vi "BuildGrid.vi"(6 "Ygoal":dbl format="%#_13g", 7 "GridParameter":dbl, 8 "Ystart":dbl format="%#_13g", 9 "Xgoal":dbl format="%#_13g", 10 "Xstart":dbl format="%#_13g") -> (0 "Nó goal":dbl[](array[numeric]), 1 "ClosedSet out":dbl[][](array[numeric]), 2 "grid out":T1, 3 "Nó start":dbl[](array[numeric]))   [LabVIEW 2016]
uses:
  Core/AI Input.ctl
  Core/AI Robot.ctl
  Intel/Functions Enum.ctl
  Intel/AttackerStates.ctl
  Core/AI Ball.ctl
  Core/Field Size.ctl
  Core/AI Judge.ctl
  Intel/Command Enum.ctl
  Util/Events/Events.ctl
  grid.ctl
  elementGrid.ctl
panel:
  in  "y pai":dbl
  in  "x pai":dbl
  in  "id":dbl
  in  "G":dbl
  in  "H":dbl
  in  "F":dbl
  in  "dy 2":dbl[](array[numeric])=[1.0, -1.0, 0.0, 0.0, 1.0, -1.0, 1.0, -1.0]
  in  "dx 2":dbl[](array[numeric])=[0.0, 0.0, 1.0, -1.0, 1.0, 1.0, -1.0, -1.0]
  in  "dy":dbl[](array[numeric])=[1.0, -1.0, 0.0, 0.0, 1.0, -1.0, 1.0, -1.0]
  in  "dx":dbl[](array[numeric])=[0.0, 0.0, 1.0, -1.0, 1.0, 1.0, -1.0, -1.0]
  in  "IA State Input":T3={"our_robots"=[], "enemy_robots"=[], "balls"=[], "geometry"={"line_width"=0, "field_length"=0, "field_width"=0, "boundary_width"=0, "referee_width"=0, "goal_width"=0, "goal_depth"=0, "goal_wall_width"=0, "center_circle_radius"=0, "defense_radius"=0, "defense_stretch"=0, "free_kick_from_defense_dist"=0, "penalty_spot_from_field_line_dist"=0, "penalty_line_from_spot_dist"=0}, "IA Judge"={"stage"="", "command"="", "our_goalie_id"=0.0, "enemy_goalie_id"=0.0, "command enum"=enum."Halt", "Time"=enum."Azul"}, "Received Timestamp"=timestamp(0 s since 1904-01-01), "Events"={"Touch"=FALSE, "Ball out"=FALSE, "id touch"=0.0, "Ball out of \nVision"=FALSE, "Ball inside \nGoalie area"=FALSE, "Robot not responding"=FALSE, "Robots responding status"=[1.0, 1.0, 1.0, 1.0, 1.0, 1.0], "Enemy Ball \nPossession"=FALSE, "Pass State"=FALSE, "id end of pass"=0.0, "Kick"=FALSE, "Id ini Possession"=0.0, "Ball Possesion"=FALSE, "Id Possesion"=0.0}}
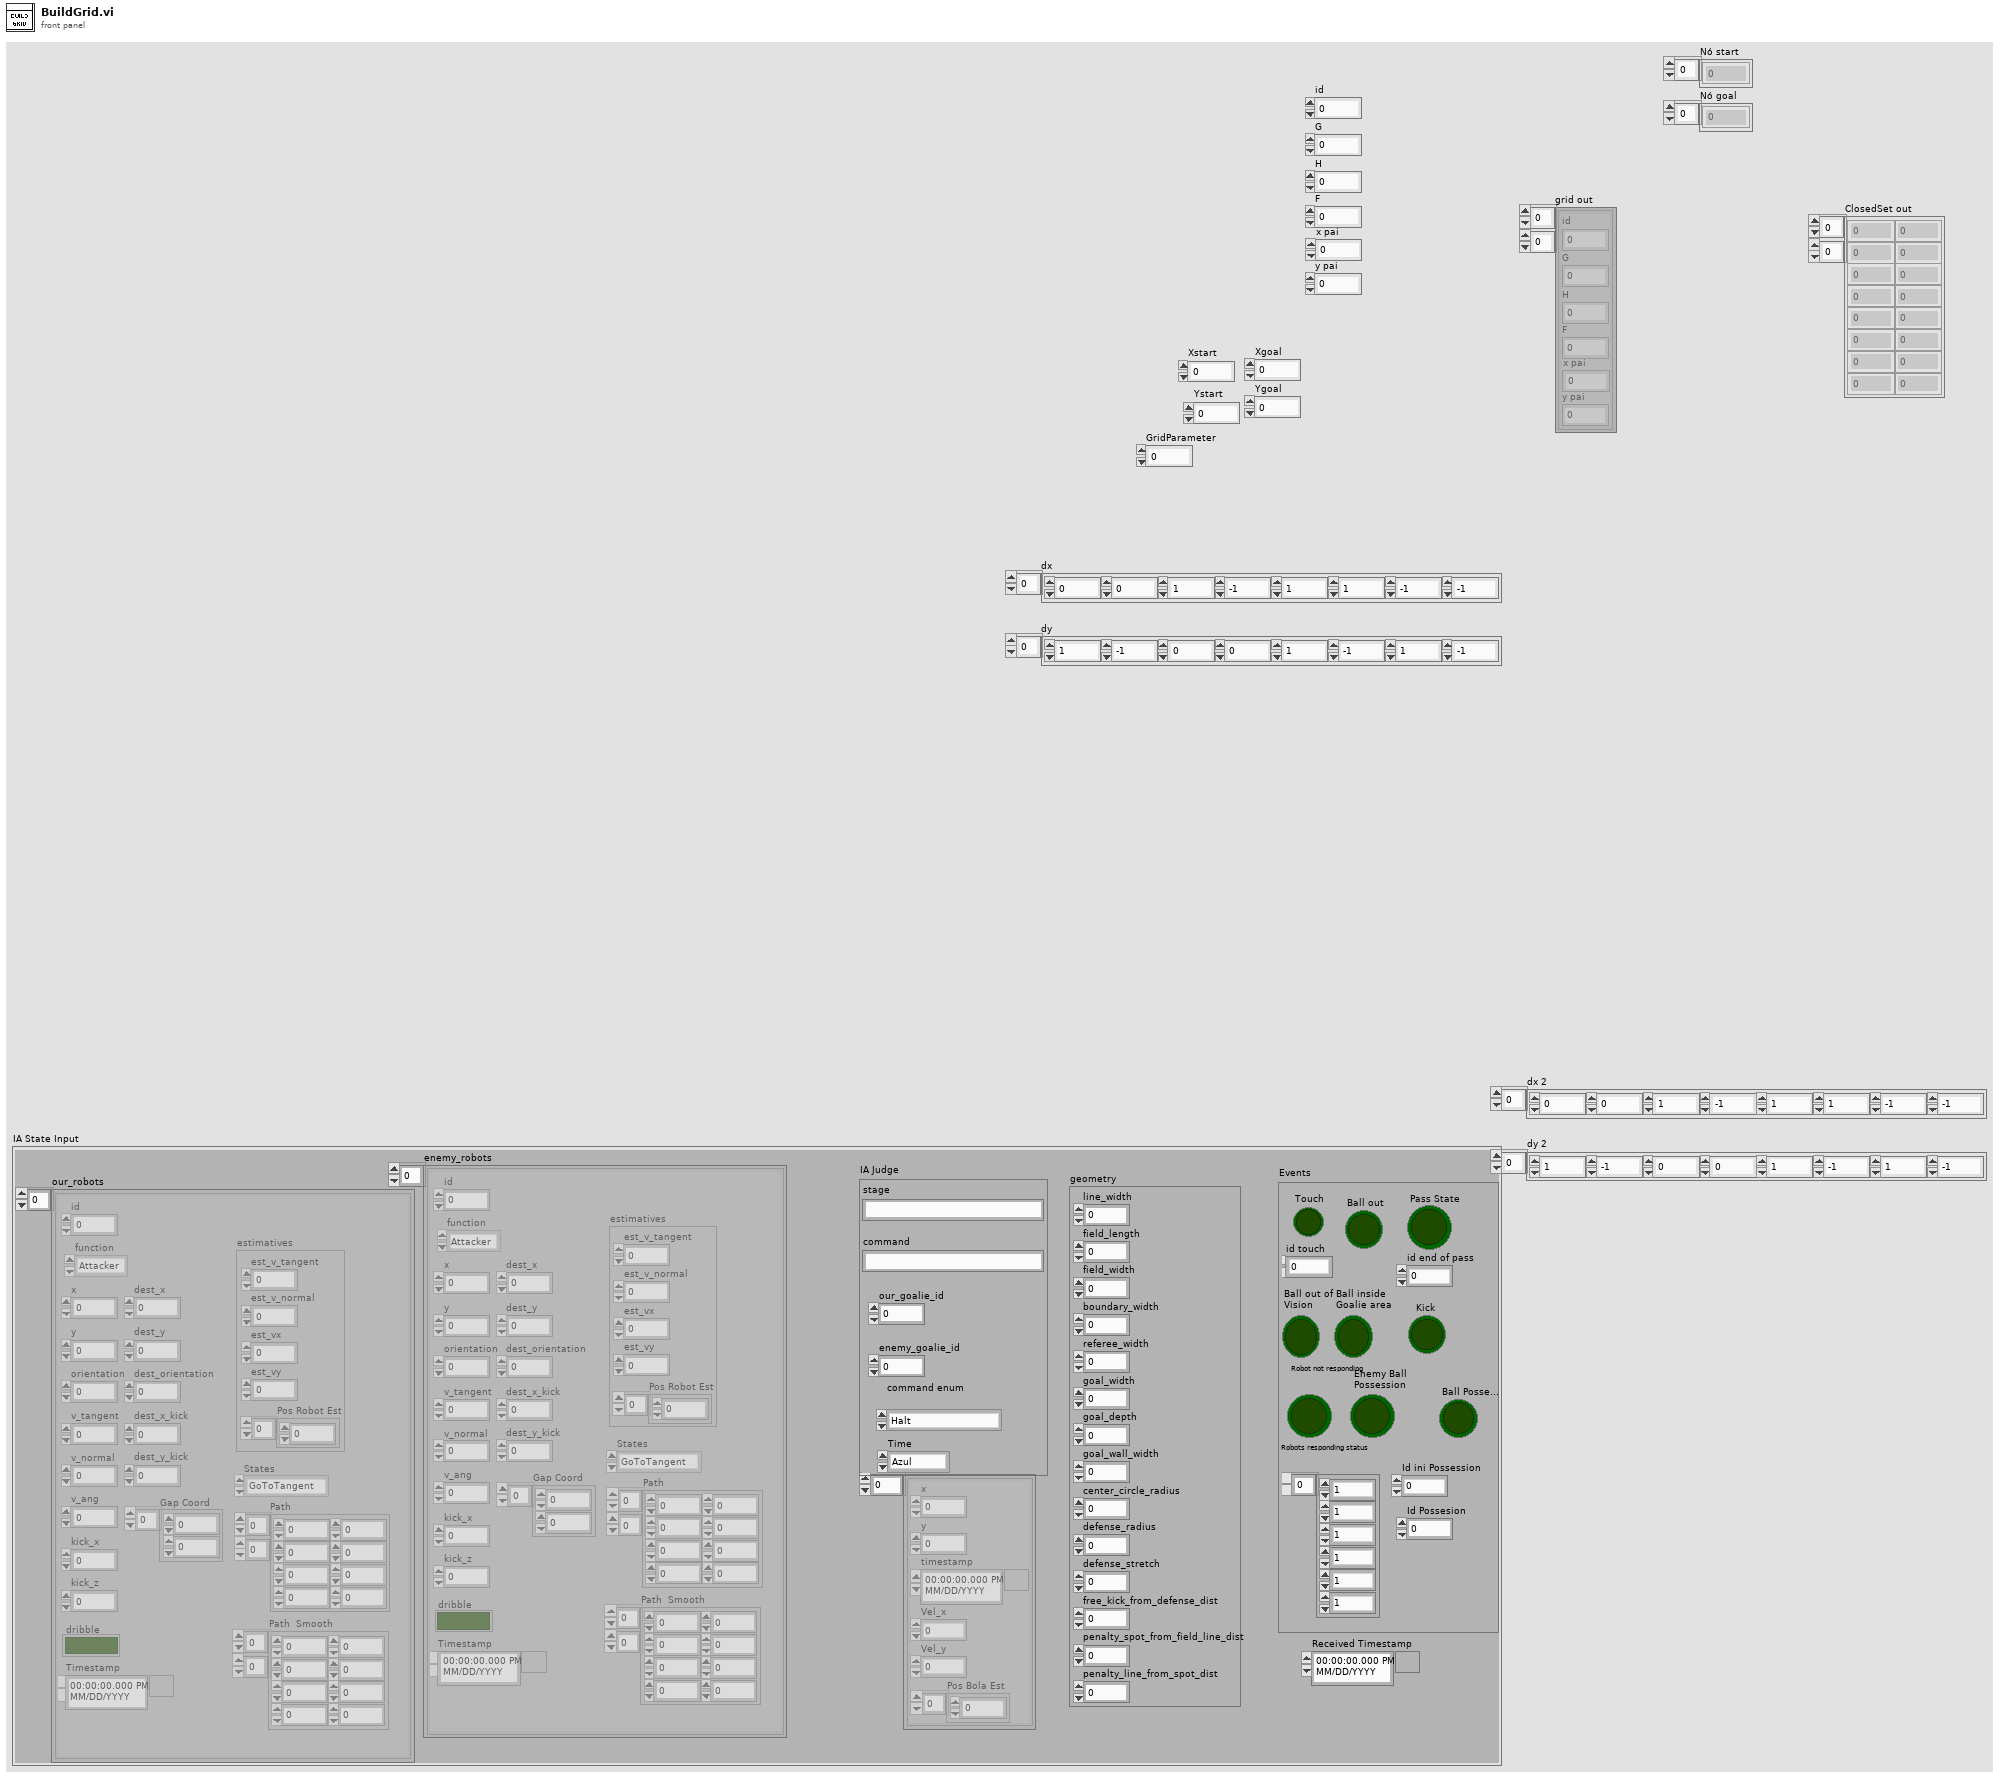
[diagram p1: front panel]
types:
  T1 = typedef "grid.ctl" = T2[][]
  T2 = typedef "elementGrid.ctl" = cluster{"id":dbl, "G":dbl, "H":dbl, "F":dbl, "x pai":dbl, "y pai":dbl}
  T3 = typedef "AI Input.ctl" = cluster{"our_robots":T4[], "enemy_robots":T4[], "balls":T7[], "geometry":T8, "IA Judge":T9, "Received Timestamp":timestamp, "Events":T11}
  T4 = typedef "AI Robot.ctl" = cluster{"id":u32, "function":T5, "x":dbl, "y":dbl, "orientation":dbl, "v_tangent":dbl, "v_normal":dbl, "v_ang":dbl, "kick_x":dbl, "kick_z":dbl, "dribble":bool, "Timestamp":timestamp, "dest_x":dbl, "dest_y":dbl, "dest_orientation":dbl, "estimatives":cluster{"est_v_tangent":dbl, "est_v_normal":dbl, "est_vx":dbl, "est_vy":dbl, "Pos Robot Est":dbl[]}, "dest_x_kick":dbl, "dest_y_kick":dbl, "Gap Coord":dbl[], "States":T6, "Path ":dbl[][], "Path  Smooth":dbl[][]}
  T5 = typedef "Functions Enum.ctl" = enum16{"Attacker", "Goalie", "Defender", "Striker", "Goto 0", "Dummy", "Kicker", "ZigZag"}
  T6 = typedef "AttackerStates.ctl" = enum16{"Pass", "GoToTangent", "BallGetting", "GoToKick", ""}
  T7 = typedef "AI Ball.ctl" = cluster{"x":dbl, "y":dbl, "timestamp":timestamp, "Vel_x":dbl, "Vel_y":dbl, "Pos Bola Est":dbl[]}
  T8 = typedef "Field Size.ctl" = cluster{"line_width":u32, "field_length":u32, "field_width":u32, "boundary_width":u32, "referee_width":u32, "goal_width":u32, "goal_depth":u32, "goal_wall_width":u32, "center_circle_radius":u32, "defense_radius":u32, "defense_stretch":u32, "free_kick_from_defense_dist":u32, "penalty_spot_from_field_line_dist":u32, "penalty_line_from_spot_dist":u32}
  T9 = typedef "AI Judge.ctl" = cluster{"stage":string, "command":string, "our_goalie_id":dbl, "enemy_goalie_id":dbl, "command enum":T10, "Time":enum16{"Azul", "Amarelo"}}
  T10 = typedef "Command Enum.ctl" = enum16{"Halt", "Stop", "Force Start", "PKA Normal Start", "Prepare Kickoff Ally", "PKE Normal Start", "Prepare Kickoff Enemy", "Prepare Penalty Ally", "PPA Normal Start", "Prepare Penalty Enemy", "PPE Normal Start", "Direct Free Enemy", "Direct Free Ally", "Indirect Free Enemy", "Indirect Free Ally", "Timeout Enemy", "Timeout Ally", "Goal Enemy", "Goal Ally", "Ball Placement Enemy", "Ball Placement Ally", "Normal Half Time", "Extra Time Break", "Extra Half Time", "None", "Post Game"}
  T11 = typedef "Events.ctl" = cluster{"Touch":bool, "Ball out":bool, "id touch":dbl, "Ball out of \nVision":bool, "Ball inside \nGoalie area":bool, "Robot not responding":bool, "Robots responding status":dbl[], "Enemy Ball \nPossession":bool, "Pass State":bool, "id end of pass":dbl, "Kick":bool, "Id ini Possession":dbl, "Ball Possesion":bool, "Id Possesion":dbl}
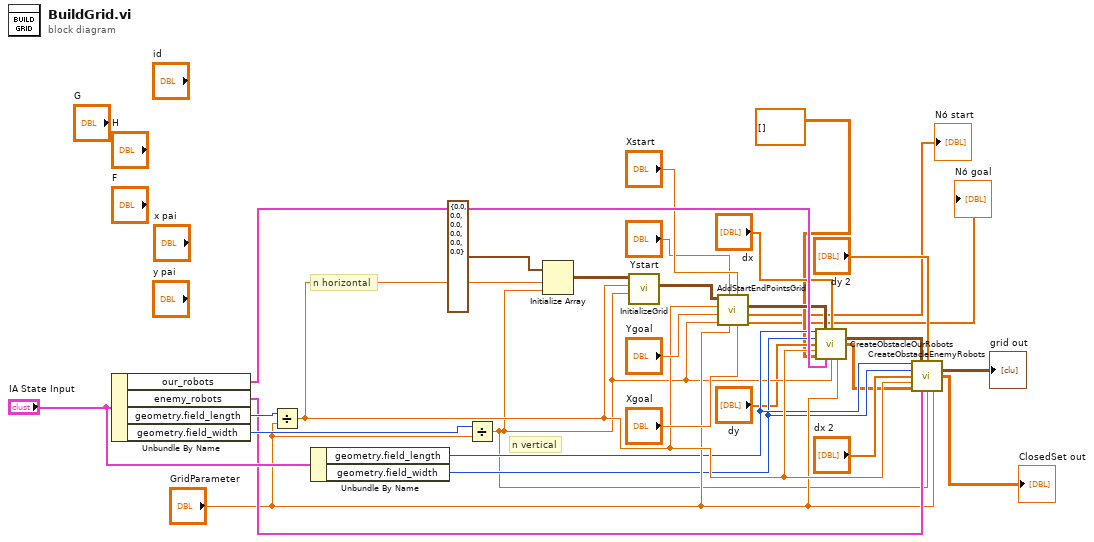
[diagram p0: block diagram]
diagram:
  # "n vertical"
  # "n horizontal"
  n1 = Unbundle By Name("IA State Input") -> ("our_robots"=w28:T4[], "enemy_robots"=w20:T4[], "geometry.field_length"=w29:u32, "geometry.field_width"=w26:u32)
  n2 = Divide(x=w29, y="GridParameter") -> (x/y=w19:dbl)
  n3 = Unbundle By Name("IA State Input") -> ("geometry.field_length"=w17:u32, "geometry.field_width"=w16:u32)
  n4 = Divide(x=w26, y="GridParameter") -> (x/y=w15:dbl)
  n5 = Initialize Array(T2 {"id"=0.0, "G"=0.0, "H"=0.0, "F"=0.0, "x pai"=0.0, "y pai"=0.0} ("element"), w19, w15) -> (w2:T2[][])
  n6 = call "InitializeGrid.vi"("n vertical"=w15, "n horizontal"=w19, "grid in"=w2) -> ("grid out"=w1:T1)  [unwired: 8 in]
  n7 = call "AddStartEndPointsGrid.vi"("Xgoal"="Xgoal", "Xstart"="Xstart", "GridParameter"="GridParameter", "Ystart"="Ystart", "n vertical"=w15, "Ygoal"="Ygoal", "n horizontal"=w19, "grid in"=w1) -> ("Nó goal"=→"Nó goal":dbl[], "Nó start"=→"Nó start":dbl[], "grid out"=w21:T1)  [unwired: 1 in]
  n8 = call "CreateObstacleOurRobots.vi"("field_length"=w17, "grid in"=w21, "dy in"="dx", "field_width"=w16, "dx in"="dy", "n horizontal"=w19, "ClosedSet in"=dbl[][] [], "our robots"=w28, "n vertical"=w15, "GridParameter"="GridParameter") -> ("grid out"=w10:T1, "ClosedSet out"=w9:dbl[][])  [unwired: 4 in]
  n9 = call "CreateObstacleEnemyRobots.vi"("field_length"=w17, "grid in"=w10, "dy in"="dy 2", "field_width"=w16, "dx in"="dx 2", "n horizontal"=w19, "ClosedSet"=w9, "enemy_robots"=w20, "n vertical"=w15, "GridParameter"="GridParameter") -> ("grid out"=→"grid out":T1, "ClosedSet out"=→"ClosedSet out":dbl[][])  [unwired: 4 in]
